vi "Receive.vi"(6 "clear_timeout_error (f)":bool, 7 "mode (standard)":T1(ring), 8 "error in (no error)":errorcluster, 10 "bufsize (548)":u32=548, 11 "Socket.UDP in":refnum<class "Socket.UDP.lvclass">) -> (0 "error out":errorcluster, 1 "bytes_read":i32, 2 "data out":string, 3 "Socket.UDP out":refnum<class "Socket.UDP.lvclass">)   [LabVIEW 2014, in "Socket.lvlib" / "Socket.UDP.lvclass"]
doc: "enum mode ignored for UDP.\n\nI32 bufsize is the maximum number of bytes to read. Default is 548 and if you wire any value other than 548 to bufsize, windows mya return an error because the function cannot read fewer bytes than are in a packet\n\nbool clear_timeout_error optional input to clear the timeout error before exiting the method. This is used when looping receive to check for loop exit conditions."
uses:
  Socket.UDP.lvclass
  Socket.UDP.lvclass/Socket.UDP.ctl
  Socket.Base/Socket.Base.lvclass/Socket.Base.ctl
  Accessors/Read udp_refnum.vi
  Socket.Base/Accessors/Read timeout.vi
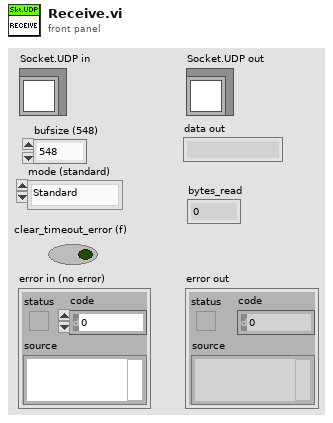
[diagram p1: front panel]
types:
  T1 = enum16{"Standard", "Buffered", "CRLF", "Immediate"}
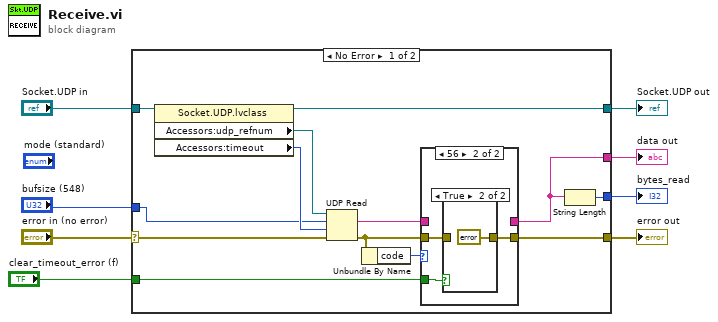
[diagram p0: block diagram]
diagram:
  n1 = case shown="No Error" "error in (no error)" {
    selector: "error in (no error)" -> [w20 w30]
    tunnel: [w9 w30] -> w7
    tunnel: [w19 w29] -> w5
    tunnel: "Socket.UDP in" -> [w21 w29]
    tunnel: "bufsize (548)" -> [w16 _]
    tunnel: [w15 _] -> w4
    tunnel: [w11 _] -> w3
    tunnel: "clear_timeout_error (f)" -> [w10 _]
    frame No Error {
      n2 = property class="Socket.UDP.lvclass"(reference=w21) -> (reference out=w19:refnum<class "Socket.UDP.lvclass">, "Accessors:udp_refnum"=w18:refnum<k16>, "Accessors:timeout"=w17:i32)  [unwired: 1 in, 1 out]
      n3 = UDP Read(connection ID=w18, max size (548)=w16, timeout ms (25000)=w17, 8:w20) -> (data out=w12:string, error out=w13:errorcluster)  [unwired: 3 out]
      n4 = Unbundle By Name(w13) -> ("code"=w14:i32)
      n5 = case shown="56" w14 {
        tunnel: w13 -> [w23 w24]
        tunnel: w12 -> [w22 _]
        tunnel: [w23 w25] -> w9
        tunnel: [w22 _] -> w11
        tunnel: w10 -> [_ w26]
        frame 0, Default {
        }
        frame 56 {
          n6 = case shown="True" w26 {
            tunnel: [w27 errorcluster {"status"=FALSE, "code"=0, "source"=""} ("error constant")] -> w25
            tunnel: w24 -> [w27 _]
            frame False {
            }
            frame True {
            }
          }
        }
      }
      n7 = String Length(string=w11) -> (length=w15:i32)
    }
    frame Error {
    }
  }
  "error out" <- w7
  "Socket.UDP out" <- w5
  "data out" <- w3
  "bytes_read" <- w4
